vi "Target Tracking.vi"() -> ()   [LabVIEW 2015]
doc: "This example shows how to track a target in an image based on a template. The user can select from three different target templates. The example can easily be modified to run from a live camera, track other targets, or track more targets. Detailed help on the example can be found in the Target Tracking Readme.html file that is included in the project."
panel:
  in  "Target Template":enum32{"Template 3", "Template 1", "Template 2"}(radio)=enum."Template 1"
  out "Input Image":T1(plugin-control)
  out "Processed Image":T1(plugin-control)
  in  "Stop (F)":bool caption="Stop"
  in  "Loop Delay (ms)":u32(slide)=200 scale=0.0..250.0
  # "1. Select a target template PRIOR to running this VI."
  # "2. Run this VI."
  # "3. Control the playback speed by adjusting the Loop Delay."
  # "See Target Tracking\nReadme.htm for more detailed information"
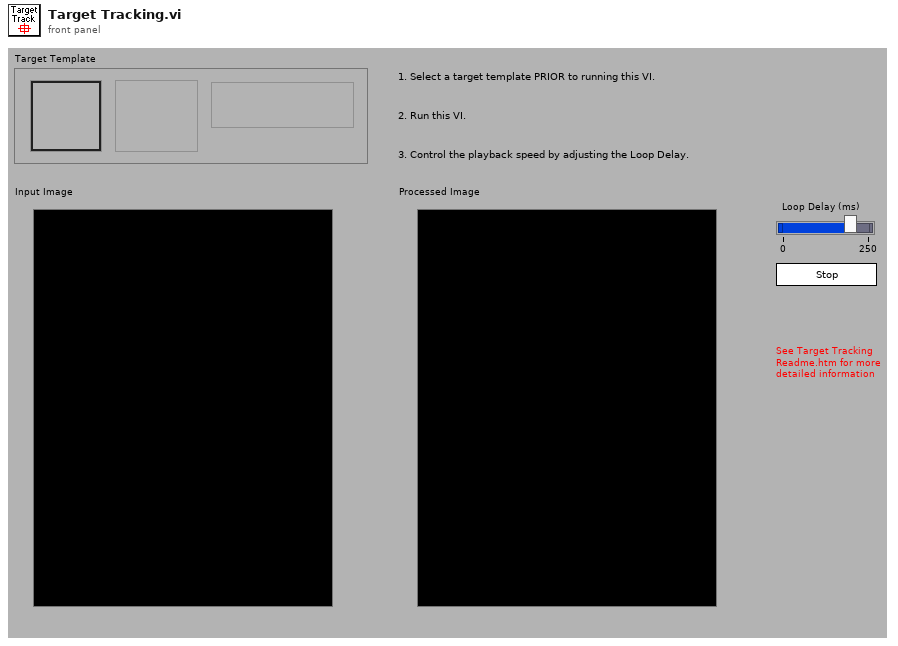
[diagram p1: front panel]
types:
  T1 = typedef "IMAQ Image.ctl" = refnum<image>
  T2 = cluster{"Position":cluster{"x":sgl, "y":sgl}, "Angle":sgl, "Scale":sgl, "Score":sgl, "Bounding Box":cluster{"x":sgl, "y":sgl}[]}[]
  T3 = typedef "ROI Descriptor" = cluster{"Global Rectangle":i32[], "Contours":cluster{"ID":enum32{"External", "Internal"}, "Type":u32, "Coordinates":i32[]}[]}
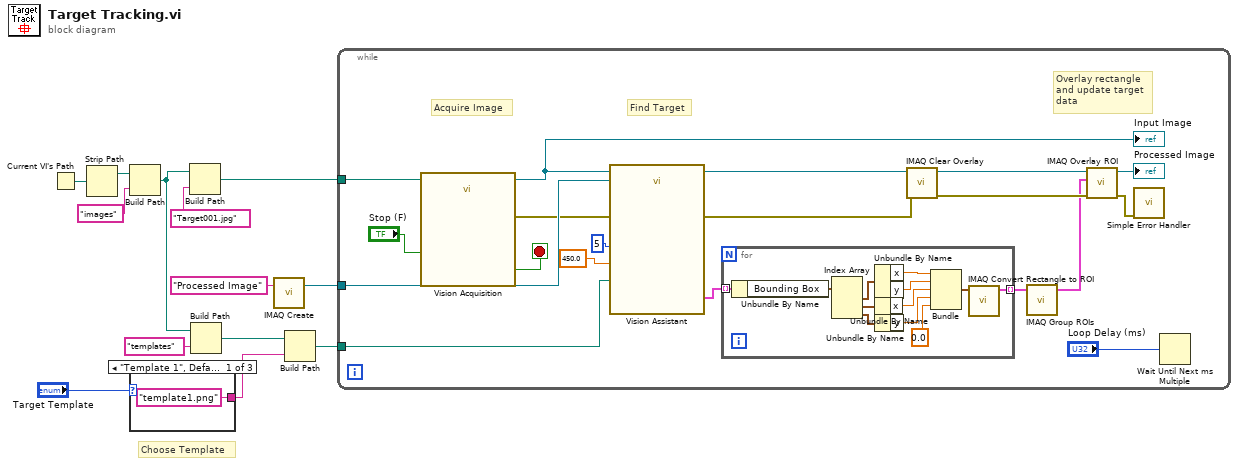
[diagram p0: block diagram]
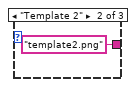
[diagram p2: hidden frame]
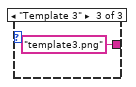
[diagram p3: hidden frame]
diagram:
  # "Choose Template"
  n1 = Current VI's Path() -> (path=w11:path)
  n2 = Strip Path(path=w11) -> (stripped path=w4:path)  [unwired: 1 out]
  n3 = Build Path(base path=w4, name or relative path="images") -> (appended path=w2:path)
  n4 = case shown="\"Template 1\", Default" "Target Template" {
    tunnel: ["template1.png" ("name or relative path") "template2.png" ("name or relative path") "template3.png" ("name or relative path")] -> w5
    frame "Template 1", Default {
    }
    frame "Template 2" {
    }
    frame "Template 3" {
    }
  }
  n5 = Build Path(base path=w2, name or relative path="Target001.jpg") -> (appended path=w8:path)
  n6 = Build Path(base path=w2, name or relative path="templates") -> (appended path=w1:path)
  n7 = call "IMAQ Create"("Image Name"="Processed Image") -> ("New Image"=w13:T1)  [unwired: 3 in, 2 out]
  n8 = Build Path(base path=w1, name or relative path=w5) -> (appended path=w7:path)
  n9 = while {
    tunnel: w13 -> [w34]
    tunnel: w8 -> [w27]
    tunnel: w7 -> [w18]
    stop <- w35 stop-if-true
    # "Overlay rectangle\nand update target\ndata"
    # "Find Target"
    # "Acquire Image"
    n10 = call "Vision Acquisition"("Image Path"=w27, "Stop (F)"="Stop (F)") -> ("Image Out"=w17:T1, "Stopped"=w35:bool, "error out"=w33:errorcluster)  [unwired: 1 in, 22 out]
    "Input Image" <- w17
    n11 = call "Vision Assistant"("Image In"=w17, "Image Dst"=w34, "Number of Matches Requested (Pattern Matching)"=5 ("Number of Matches Requested (Pattern Matching 1)"), "Minimum Match Score (Pattern Matching)"=sgl 450.0 ("Minimum Match Score"), "Template File Path (Pattern Matching)"=w18, "error in"=w33) -> ("Image Out"=w32:T1, "Matches (Pattern Matching)"=w22:T2, "error out"=w30:errorcluster)  [unwired: 19 out]
    n12 = for {
      tunnel: w22 -> [w47] mode=indexing
      tunnel: [w38] -> w21 mode=indexing
      n13 = Unbundle By Name(w47) -> ("Bounding Box"=w46:cluster{"x":sgl, "y":sgl}[])
      n14 = Index Array(array=w46) -> (element #1=w45:cluster{"x":sgl, "y":sgl}, element #2=w44:cluster{"x":sgl, "y":sgl}, element #3=w37:cluster{"x":sgl, "y":sgl})  [unwired: 3 in]
      n15 = Unbundle By Name(w45) -> ("x"=w43:sgl, "y"=w42:sgl)
      n16 = Unbundle By Name(w44) -> ("x"=w41:sgl)
      n17 = Unbundle By Name(w37) -> ("y"=w36:sgl)
      n18 = Bundle("x"=w43, "y"=w42, "x"=w41, "y"=w36, 0.0) -> (w39:cluster{"x":sgl, "y":sgl, "x":sgl, "y":sgl, dbl})  [unwired: 1 out]
      n19 = call "IMAQ Convert Rectangle to ROI"("Rectangle"=w39) -> ("ROI Descriptor"=w38:T3)  [unwired: 1 in, 8 out]
    }
    n20 = call "IMAQ Clear Overlay"("error in (no error)"=w30, "Image"=w32) -> ("error out"=w29:errorcluster, "Image Out"=w19:T1)  [unwired: 1 in, 7 out]
    n21 = call "IMAQ Group ROIs"("ROI Descriptors"=w21) -> ("ROI Descriptor out"=w20:T3)  [unwired: 1 in, 3 out]
    n22 = call "IMAQ Overlay ROI"("error in (no error)"=w29, "ROI Descriptor"=w20, "Image"=w19) -> ("error out"=w25:errorcluster, "Image Out"=→"Processed Image":T1)  [unwired: 3 in, 4 out]
    n23 = call <vilib>:"Simple Error Handler.vi"("error in (no error)"=w25) -> ()  [unwired: 1 in, 8 out]
    n24 = Wait Until Next ms Multiple(millisecond multiple="Loop Delay (ms)") -> ()  [unwired: 1 out]
  }
